vi "HFRR ADV v13.vi"() -> ()   [LabVIEW 2025] (continued)
                        n2641 = property on="Humidity ( %RH )" class="WFChart (strict)"("History Data"=w3931) -> ()  [unwired: 2 in, 2 out]
                        n2642 = property on="Stroke ( mm )" class="WFChart (strict)"("History Data"=w3932) -> ()  [unwired: 2 in, 2 out]
                        n2643 = property on="Temperature ( Deg C )" class="WFChart (strict)"("History Data"=w3931) -> ()  [unwired: 2 in, 2 out]
                        n2644 = property on="Service Password Log" class="Str"("Visible"=w3933) -> ()  [unwired: 2 in, 2 out]
                        n2645 = property on="Password 3" class="Clust (strict)"("Visible"=w3933) -> ()  [unwired: 2 in, 2 out]
                      }
                    }
                    "TEST FILE NAM,E SAVED" <- TRUE ("TEST FILE NAM,E SAVED")
                  }
                }
              }
            }
          }
        }
        n2646 = case shown="True" w3205 {
          frame False {
            n2647 = local write "tfalg"(0.0 ("tfalg")) -> ()
          }
          frame True {
            n2648 = local read "tfalg"() -> (w3350:dbl)
            n2649 = Equal?(x=w3350, y=0.0) -> (x = y?=w3351:bool)
            n2650 = case shown="True" w3351 {
              frame False {
              }
              frame True {
                n2651 = local read "Total No. of Tests"() -> (w3354:dbl)
                n2652 = local write "tfalg"(1.0 ("tfalg")) -> ()
                n2653 = local write "acq 2"(FALSE ("acq 2")) -> ()
                n2654 = Wait (ms)(milliseconds to wait=u32 200) -> ()  [unwired: 1 out]
                n2655 = Increment(x=w3354) -> (x+1=w3353:dbl)
                n2656 = local write "Total No. of Tests"(w3353) -> ()
              }
            }
          }
        }
        n2657 = local write "Test \nStatus"(w3211) -> ()
        n2658 = local write "st enable"(w3211) -> ()
        n2659 = local write "PWR"(w3211) -> ()
        n2660 = local write "Save"(w3211) -> ()
        n2661 = local read "Main Tab"() -> (w3168:T2)
        n2662 = case shown="True" w3192 {
          tunnel: [FALSE ("RUN") TRUE ("RUN")] -> w3191
          tunnel: [_ 1] -> w3184
          frame False {
          }
          frame True {
          }
        }
        n2663 = In Range and Coerce(upper limit=w3199, x=w3172, lower limit=w3198) -> (In Range?=w3190:bool)  [unwired: 1 out]
        n2664 = In Range and Coerce(upper limit=w3196, x=w3171, lower limit=w3197) -> (In Range?=w3188:bool)  [unwired: 1 out]
        n2665 = case shown="True" w3204 {
          frame False {
            n2666 = local read "Rt 3"() -> (w3332:bool)
            n2667 = case shown="True" w3332 {
              frame False {
              }
              frame True {
                n2668 = local write "Rt 3"(FALSE ("Rt 3")) -> ()
                n2669 = local write "Json End Flg"(TRUE ("Upld AR 2")) -> ()
              }
            }
            "Rt" <- TRUE ("Rt")
            "Rt 2" <- FALSE ("Rt")
          }
          frame True {
            n2670 = local read "Rt"() -> (w3339:bool)
            n2671 = local write "Rt 2"(TRUE ("Rt 2")) -> ()
            n2672 = case shown="True" w3339 {
              frame False {
              }
              frame True {
                w3340 = TRUE ("Upld AR 2")
                n2673 = local write "Rt"(FALSE ("Rt")) -> ()
                n2674 = local write "Upld AR"(w3340) -> ()
                n2675 = local write "Json St Flg"(w3340) -> ()
              }
            }
            "Rt 3" <- TRUE ("Rt 3")
          }
        }
        n2676 = case shown="True" w3190 {
          tunnel: [FALSE ("RUN") TRUE ("RUN")] -> w3189
          tunnel: [_ 2] -> w3183
          frame False {
          }
          frame True {
          }
        }
        n2677 = case shown="True" w3188 {
          tunnel: [FALSE ("RUN") TRUE ("RUN")] -> w3187
          tunnel: [_ 3] -> w3182
          frame False {
          }
          frame True {
          }
        }
        n2678 = case shown="\"Acquire\"" w3168 {
          tunnel: w3170 -> [_ w3401]
          frame Default {
            w3400 = 0.0 ("output")
            n2679 = local write "PID-out"(w3400) -> ()
            n2680 = local write "Frequency ( Hz )"(w3400) -> ()
          }
          frame "Acquire" {
            n2681 = stacked-sequence {
              frame #0 {
                n2682 = local read "Auto Start Test"() -> (w3403:bool)
                n2683 = case shown="True" w3403 {
                  tunnel: "RUN" -> [w3424 w3427]
                  tunnel: [w3424 w3426] -> w3404
                  frame False {
                  }
                  frame True {
                    n2684 = local read "Auto Start Temp"() -> (w3425:bool)
                    n2685 = Or(x=w3427, y=w3425) -> (x .or. y?=w3426:bool)
                  }
                }
                n2686 = local read "clk"() -> (w3423:dbl)
                n2687 = local read "Save"() -> (w3419:bool)
                n2688 = Equal?(x=w3423, y=0.0) -> (x = y?=w3420:bool)
                n2689 = And(x=w3420, y=w3419) -> (x .and. y?=w3421:bool)
                n2690 = Not(x="Engage") -> (.not. x?=w3410:bool)
                n2691 = case shown="True" w3404 {
                  tunnel: [w3435 w3453] -> w3406
                  frame False {
                    w3435 = 0.0
                    n2692 = local read "Auto Start Test"() -> (w3431:bool)
                    n2693 = local write "Reinit PID"(TRUE) -> ()
                    n2694 = local write "Start Time"(TRUE ("Start Time")) -> ()
                    n2695 = property on="Stroke" class="DigNum (strict)"("Visible"=TRUE) -> ()  [unwired: 2 in, 2 out]
                    n2696 = property on="Stroke 2" class="DigNum (strict)"("Visible"=FALSE) -> ()  [unwired: 2 in, 2 out]
                    n2697 = case shown="False" w3431 {
                      frame False {
                        n2698 = property on="Heater Button" class="Bool (strict)"("DisabledEnum"=T16."Enabled" ("Disabled")) -> ()  [unwired: 2 in, 2 out]
                        n2699 = property on="Humidity" class="Bool (strict)"("DisabledEnum"=T16."Enabled" ("Disabled")) -> ()  [unwired: 2 in, 2 out]
                      }
                      frame True {
                      }
                    }
                    n2700 = case shown="False" "TestCompFlg" {
                      frame False {
                        n2701 = local read "StartFlg"() -> (w3441:bool)
                        n2702 = case shown="True" w3441 {
                          frame False {
                          }
                          frame True {
                            n2703 = flat-sequence {
                              frame #0 {
                                n2704 = local read "EVENT LOG"() -> (w3443:string)
                                n2705 = call "Event Log.vi"("Content"="Test was interrupted", "EVENT LOG"=w3443) -> ("EVENT LOG"=w3444:string)  [unwired: 8 in, 1 out]
                                n2706 = local write "EVENT LOG"(w3444) -> ()
                              }
                              frame #1 {
                                w3445 = FALSE ("StartFlg")
                                n2707 = local write "Heater Button"(w3445) -> ()
                                n2708 = local write "StartFlg"(w3445) -> ()
                                n2709 = local write "Humidity"(w3445) -> ()
                              }
                            }
                          }
                        }
                      }
                      frame True {
                      }
                    }
                    n2710 = local write "String 14"("Test will autostart once parameters reach the set value." ("String 14")) -> ()
                    n2711 = local write "Old Pid Val"(w3435) -> ()
                  }
                  frame True {
                    n2712 = property on="Stroke 2" class="DigNum (strict)"("Visible"=TRUE) -> ()  [unwired: 2 in, 2 out]
                    n2713 = property on="Stroke" class="DigNum (strict)"("Visible"=FALSE) -> ()  [unwired: 2 in, 2 out]
                    n2714 = property on="STOP 2" class="Bool (strict)"("Disabled"=u8 2) -> ()  [unwired: 2 in, 2 out]
                    n2715 = local write "String 14"(" Running....." ("String 14")) -> ()
                    n2716 = property on="Heater Button" class="Bool (strict)"("DisabledEnum"=T16."Disabled and Grayed Out" ("Disabled")) -> ()  [unwired: 2 in, 2 out]
                    n2717 = property on="Humidity" class="Bool (strict)"("DisabledEnum"=T16."Disabled and Grayed Out" ("Disabled")) -> ()  [unwired: 2 in, 2 out]
                    n2718 = local read "PID Ref"() -> (w3464:bool)
                    n2719 = case shown="True" w3464 {
                      tunnel: [w3470 w3486] -> w3463
                      frame False {
                        n2720 = local read "Old Pid Val"() -> (w3470:dbl)
                      }
                      frame True {
                        n2721 = local read "Set Hz"() -> (w3479:dbl)
                        n2722 = local read "Frequency"() -> (w3490:dbl)
                        n2723 = Add(x=w3479, y=10.0) -> (x+y=w3488:dbl)
                        n2724 = Add(x=w3479, y=-10.0 ("Offset")) -> (x+y=w3497:dbl)
                        n2725 = Add(x=w3479, y=-10.0) -> (x+y=w3489:dbl)
                        n2726 = In Range and Coerce(upper limit=w3488, x=w3490, lower limit=w3489) -> (coerced(x)=w3478:dbl)  [unwired: 1 out]
                        n2727 = Or(x="Reinit PID", y="Reinit PID") -> (x .or. y?=w3487:bool)
                        n2728 = Multiply(x=w3497, y=0.1 ("Gain")) -> (x*y=w3476:dbl)
                        n2729 = local read "Elapsed time"() -> (w3483:dbl)
                        n2730 = local read "SPEED OUT:"() -> (w3498:dbl)
                        n2731 = Add(x=w3476, y=1.5) -> (x+y=w3474:dbl)
                        n2732 = call-poly <vilib>:"PID.vi"("reinitialize? (F)"=w3487, "output range"=cluster{"output high":dbl, "output low":dbl} {"output high"=1.0, "output low"=-1.0}, "PID gains"=T13 {"proportional gain (Kc)"=0.0005, "integral time (Ti, min)"=0.001, "derivative time (Td, min)"=0.0} ("Motor PID"), "process variable"=w3478, "setpoint"=w3479) -> ("output"=w3477:dbl)  [unwired: 5 in, 1 out]
                        n2733 = Multiply(x=w3474, y=w3498) -> (x*y=w3473:dbl)
                        n2734 = Greater?(x=w3483, y=0.05) -> (0:w3482:bool)
                        n2735 = case shown="True" w3482 {
                          tunnel: w3477 -> [_ w3500]
                          tunnel: [0.0 ("output") w3500] -> w3480
                          frame False {
                          }
                          frame True {
                            n2736 = local write "Reinit PID"(FALSE ("Reinit PID")) -> ()
                          }
                        }
                        n2737 = Multiply(x=w3473, y=0.8) -> (x*y=w3472:dbl)
                        n2738 = Add(x=w3472, y=w3480) -> (x+y=w3485:dbl)
                        n2739 = flat-sequence {
                          tunnel: [w3503] -> w3486
                          tunnel: w3485 -> [w3503]
                          frame #0 {
                            n2740 = local write "PID Ref"(FALSE ("PID Ref")) -> ()
                          }
                        }
                      }
                    }
                    "Old Pid Val" <- w3463
                    n2741 = case shown="True" "Start Time" {
                      selector: "Start Time" -> [_ w3466]
                      frame False {
                      }
                      frame True {
                        n2742 = Not(x=w3466) -> (.not. x?=w3465:bool)
                        n2743 = local write "Start Time"(w3465) -> ()
                        n2744 = local read "EVENT LOG"() -> (w3467:string)
                        n2745 = call "Event Log.vi"("Content"="Test in progress", "EVENT LOG"=w3467) -> ("EVENT LOG"=w3469:string)  [unwired: 8 in, 1 out]
                        n2746 = local write "EVENT LOG"(w3469) -> ()
                      }
                    }
                    n2747 = local read "Set Hz"() -> (w3460:dbl)
                    n2748 = call <vilib>:"Uniform White Noise Waveform.vi"() -> ("signal out"=w3459:waveform(dbl))  [unwired: 10 in, 1 out]
                    n2749 = local read "Freq"() -> (w3452:dbl)
                    n2750 = Add(x=w3460, y=w3459) -> (x+y=w3458:waveform(dbl))
                    n2751 = Multiply(x=w3458, y=ext 0.1) -> (x*y=w3454:waveform(ext))
                    n2752 = Multiply(x=w3452, y=0.9) -> (x*y=w3455:dbl)
                    n2753 = Add(x=w3454, y=w3455) -> (x+y=w3453:waveform(ext))
                    "StartFlg" <- TRUE ("StartFlg")
                  }
                }
                n2754 = case shown="True" w3421 {
                  frame False {
                  }
                  frame True {
                    n2755 = local write "clk"(10.0 ("clk")) -> ()
                    n2756 = Get Date/Time In Seconds() -> (seconds since 1Jan1904=w3506:timestamp)
                    n2757 = To Double Precision Float(number=w3506) -> (double precision float=w3504:dbl)
                    n2758 = local write "acq timer"(w3504) -> ()
                    n2759 = local write "act save time"(w3504) -> ()
                  }
                }
                n2760 = call "Elapsed Time"("Time Target (s)"="Countdown", "Reset"=w3410) -> ("Elapsed Time (s)"=w3415:dbl, "Time has Elapsed"=w3413:bool)  [unwired: 10 in, 6 out]
                "Countdown 2" <- w3415
                n2761 = Subtract(x=w3415, y=2.0) -> (x-y=w3418:dbl)
                n2762 = Less?(x=w3418, y="Countdown") -> (x < y?=w3416:bool)
                n2763 = And(x=w3416, y=w3413) -> (x .and. y?=w3412:bool)
                n2764 = case shown="True" w3412 {
                  frame False {
                  }
                  frame True {
                    (unwired) dbl[] [] ("History Data")
                    n2765 = local write "Engage"(FALSE ("Engage")) -> ()
                    n2766 = local write "RUN"(TRUE ("RUN")) -> ()
                    n2767 = local read "Humidity ( %RH )"() -> (→"Rh Before":dbl)
                  }
                }
                n2768 = local read "Test \nStatus"() -> (w3408:bool)
                n2769 = Select(t=w3406, s=w3408, f=0.0) -> (s? t:f=w3407:dbl)
                n2770 = local write "Frequency ( Hz )"(w3407) -> ()
                n2771 = local write "Freq"(w3407) -> ()
              }
              frame #1 {
                w3529 = 1000000.0 ("x")
                # "Elapsed time\ncof\nstroke\nAir temp\nTemp\nHumidity"
                # "acq timer\n\nact save time"
                # "convert to microseconds"
                n2772 = local read "COUNT"() -> (w3512:i32)
                n2773 = local read "Rate"() -> (w3525:dbl)
                n2774 = Divide(x=w3529, y=w3525) -> (x/y=w3530:dbl)
                n2775 = Greater Or Equal?(x=w3512, y=250) -> (x >= y?=w3511:bool)
                n2776 = Get Date/Time In Seconds() -> (seconds since 1Jan1904=w3532:timestamp)
                n2777 = case shown="True" w3511 {
                  frame False {
                    n2778 = local read "COUNT"() -> (w3533:i32)
                    n2779 = Increment(x=w3533) -> (x+1=w3534:i32)
                    n2780 = local write "COUNT"(w3534) -> ()
                  }
                  frame True {
                    n2781 = local write "COUNT"(0 ("COUNT")) -> ()
                  }
                }
                n2782 = local read "Samplingtime 2"() -> (w3510:dbl)
                n2783 = local read "act save time"() -> (w3527:dbl)
                n2784 = Divide(x=w3530, y=w3529) -> (x/y=w3528:dbl)
                n2785 = To Double Precision Float(number=w3532) -> (double precision float=w3521:dbl)
                n2786 = Add(x=w3527, y=w3510) -> (x+y=w3526:dbl)
                n2787 = local read "acq timer"() -> (w3531:dbl)
                n2788 = local read "COUNT"() -> (w3514:i32)
                n2789 = Greater Or Equal?(x=w3521, y=w3526) -> (x >= y?=w3509:bool)
                n2790 = Multiply(x=w3528, y=w3514) -> (x*y=w3520:dbl)
                n2791 = Subtract(x=w3521, y=w3531) -> (x-y=w3523:dbl)
                n2792 = local read "Save"() -> (w3524:bool)
                n2793 = Add(x=w3523, y=w3520) -> (x+y=w3507:dbl)
                "Elapsed time 3" <- w3507
                n2794 = And(x=w3509, y=w3524) -> (x .and. y?=w3522:bool)
                n2795 = Divide(x=w3507, y=60.0) -> (x/y=w3518:dbl)
                n2796 = local read "Test \nStatus"() -> (w3508:bool)
                n2797 = local read "clk"() -> (w3515:dbl)
                n2798 = Equal?(x=w3515, y=10.0) -> (x = y?=w3517:bool)
                n2799 = case shown="True" w3522 {
                  tunnel: w3521 -> [_ w3636]
                  tunnel: [FALSE ("Boolean 2") TRUE ("Boolean 2")] -> _
                  frame False {
                  }
                  frame True {
                    w3583 = ";" ("Substring")
                    # "Pid out/\nFreq response value"
                    n2800 = local write "act save time"(w3636) -> ()
                    n2801 = local read "FILE"() -> (w3577:string)
                    n2802 = call "file check.vi"("file name in"=w3577) -> ("error out"=w3580:errorcluster, "file name out"=w3575:string)  [unwired: 9 in]
                    n2803 = call "FILE PATH CREATION.vi"("error in"=w3580, "FILE NAME :"=w3575) -> ("FILE OUT"=w3578:path)  [unwired: 8 in, 1 out]
                    n2804 = Concatenate Strings(w3575, ".dgf" ("Substring")) -> (w3579:string)
                    n2805 = local read "Set Strk"() -> (w3607:dbl)
                    n2806 = local read "Stroke"() -> (w3598:dbl)
                    n2807 = local read "FF 2"() -> (→"Frictional Force ( N )" →"Frictional Force ( N )":dbl)
                    n2808 = Build Path(base path=w3578, name or relative path=w3579) -> (appended path=w3574:path)
                    n2809 = Subtract(x=w3598, y=w3607) -> (x-y=w3604:dbl)
                    n2810 = local read "COF 2"() -> (w3589:dbl)
                    "cof" <- w3589
                    "Coefficient of Friction" <- w3589
                    "COF 4" <- w3589
                    "Coefficient of Friction" <- w3589
                    n2811 = Multiply(x=w3604, y=0.05) -> (x*y=w3606:dbl)
                    n2812 = local read "TEMP"() -> (w3593:dbl)
                    "Temp" <- w3593
                    "Temperature ( Deg C )" <- w3593
                    n2813 = Add(x=w3606, y=w3607) -> (x+y=w3587:dbl)
                    "Stroke Ln" <- w3587
                    "Disp" <- w3587
                    n2814 = local read "ecr"() -> (w3590:dbl)
                    "Electrical Contact Resistance ( % )" <- w3590
                    n2815 = local read "Humidity ( %RH )"() -> (w3592:dbl)
                    "Humidity ( %RH )" <- w3592
                    "Humidity ( %RH )" <- w3592
                    n2816 = local read "Frequency ( Hz )"() -> (w3600:dbl)
                    n2817 = local read "Elapsed time"() -> (w3629:dbl)
                    n2818 = disable-structure shown="Disabled" {
                      frame Disabled {
                        n2819 = local read "ecr 3"() -> ()  [unwired: 1 in]
                      }
                      frame Enabled {
                      }
                    }
                    n2820 = local read "AIR TEMP"() -> (w3597:dbl)
                    n2821 = local read "PID-out"() -> (w3603:dbl)
                    n2822 = local write "Temperature ( Deg C )"(w3593) -> ()
                    n2823 = Number To Fractional String(number=w3587, width (-)=i16 9 ("precision (6)"), precision (6)=i16 6) -> (F-format string=w3622:string)  [unwired: 1 in]
                    n2824 = Number To Fractional String(number=w3597, width (-)=i16 9 ("precision (6)"), precision (6)=i16 3) -> (F-format string=w3621:string)  [unwired: 1 in]
                    n2825 = Number To Fractional String(number=w3593, width (-)=i16 9 ("precision (6)"), precision (6)=i16 3) -> (F-format string=w3618:string)  [unwired: 1 in]
                    n2826 = Number To Fractional String(number=w3592, width (-)=i16 9 ("precision (6)"), precision (6)=i16 3) -> (F-format string=w3615:string)  [unwired: 1 in]
                    n2827 = Number To Fractional String(number=w3590, width (-)=i16 9 ("precision (6)"), precision (6)=i16 3) -> (F-format string=w3612:string)  [unwired: 1 in]
                    n2828 = Number To Fractional String(number=w3603, width (-)=i16 9 ("precision (6)"), precision (6)=i16 3) -> (F-format string=w3608:string)  [unwired: 1 in]
                    n2829 = Number To Fractional String(number=w3600, width (-)=i16 9 ("precision (6)"), precision (6)=i16 3) -> (F-format string=w3599:string)  [unwired: 1 in]
                    n2830 = Number To Fractional String(number=w3589, width (-)=i16 9 ("precision (6)"), precision (6)=i16 6) -> (F-format string=w3630:string)  [unwired: 1 in]
                    n2831 = Number To Fractional String(number=w3629, width (-)=i16 14 ("precision (6)"), precision (6)=i16 3) -> (F-format string=w3631:string)  [unwired: 1 in]
                    n2832 = Bundle("y"=1.02, w3587, "y"=0.98) -> (w3591:cluster{"y":dbl, dbl, "y":dbl})  [unwired: 1 in]
                    n2833 = Number To Fractional String(number="Ambient Humidity :", width (-)=i16 9 ("precision (6)"), precision (6)=i16 6) -> (F-format string=w3581:string)  [unwired: 1 in]
                    n2834 = local read "RUN"() -> (w3588:bool)
                    n2835 = case shown="True" w3588 {
                      tunnel: w3591 -> [_ w3641]
                      tunnel: w3587 -> [_ w3640]
                      tunnel: w3587 -> [_ w3639]
                      tunnel: w3587 -> [_ w3638]
                      frame False {
                      }
                      frame True {
                        "Stroke ( mm )" <- w3641
                        "Stroke ( mm )" <- w3641
                        "Stroke 4" <- w3640
                        "Stroke 3" <- w3639
                        "Stroke 2" <- w3638
                      }
                    }
                    n2836 = Concatenate Strings(w3631, w3583, w3630, w3583, w3622, w3583, w3621, w3583, w3618, w3583, w3615, w3583, w3612, w3583, w3608, w3583, w3599, w3583, w3581, "\r") -> (w3628:string)
                    n2837 = call <vilib>:"Write Characters To File.vi"("append to file? (new file:F)"=TRUE, "character string"=w3628, "file path (dialog if empty)"=w3574) -> ()  [unwired: 2 in, 1 out]
                    "refresh flag" <- TRUE ("refresh flag")
                  }
                }
                n2838 = case shown="True" w3508 {
                  tunnel: w3518 -> [_ w3544]
                  tunnel: w3523 -> [_ w3554]
                  tunnel: [0.0 w3550] -> _
                  tunnel: w3517 -> [_ w3549]
                  tunnel: [0.0 w3548] -> _
                  tunnel: w3507 -> [_ w3548]
                  tunnel: w3521 -> [w3537 _]
                  frame False {
                    n2839 = local write "acq timer"(w3537) -> ()
                    n2840 = local write "Test Duration Status"(0.0 ("Test Duration Status")) -> ()
                  }
                  frame True {
                    n2841 = local read "Set Hz"() -> (w3551:dbl)
                    n2842 = local write "Elapsed time"(w3544) -> ()
                    n2843 = local read "test time"() -> (w3543:dbl)
                    n2844 = Multiply(x=w3554, y=w3551) -> (x*y=w3553:dbl)
                    n2845 = case shown="False" w3549 {
                      tunnel: w3553 -> [w3555 _]
                      tunnel: [w3555 1.0] -> w3550
                      frame False {
                        n2846 = local write "Cycles elapsed"(w3555) -> ()
                      }
                      frame True {
                      }
                    }
                    n2847 = Greater?(x=w3544, y=w3543) -> (0:w3552:bool)
                    n2848 = Subtract(x=w3543, y=w3544) -> (x-y=w3542:dbl)
                    "time" <- w3542
                    n2849 = Multiply(x=w3542, y=60.0) -> (x*y=w3541:dbl)
                    n2850 = local write "Time Remaining"(w3541) -> ()
                    n2851 = local write "Remaining Time"(w3541) -> ()
                    n2852 = case shown="True" w3552 {
                      frame False {
                      }
                      frame True {
                        w3557 = T16."Enabled" ("Disabled")
                        w3561 = "" ("FILE")
                        w3562 = TRUE ("Visible")
                        n2853 = local write "Humidity"(FALSE ("Humidity")) -> ()
                        n2854 = local write "RUN"(FALSE ("OK Button 2")) -> ()
                        n2855 = local write "Heater Button"(FALSE ("Heater Button")) -> ()
                        n2856 = local write "Auto Start Test"(FALSE ("Auto Start Test")) -> ()
                        n2857 = local write "TestCompFlg"(TRUE ("StpFlg")) -> ()
                        n2858 = local read "Humidity ( %RH )"() -> (→"Rh After":dbl)
                        n2859 = property on="STOP 2" class="Bool (strict)"("Disabled"=u8 0) -> ()  [unwired: 2 in, 2 out]
                        n2860 = local read "EVENT LOG"() -> (w3567:string)
                        n2861 = call "Event Log.vi"("Content"="Test Completed", "EVENT LOG"=w3567) -> ("EVENT LOG"=w3566:string)  [unwired: 8 in, 1 out]
                        n2862 = property on="RUN" class="Bool (strict)"("Visible"=w3562) -> ()  [unwired: 2 in, 2 out]
                        n2863 = property on="Auto Start Test" class="Bool (strict)"("Visible"=w3562) -> ()  [unwired: 2 in, 2 out]
                        n2864 = local write "Batch Ref Num :"(w3561) -> ()
                        n2865 = local write "FILE"(w3561) -> ()
                        n2866 = local write "EVENT LOG"(w3566) -> ()
                        n2867 = local write "TEST FILE NAM,E SAVED"(FALSE ("TEST FILE NAM,E SAVED")) -> ()
                        n2868 = local write "Fuel Discription :"(w3561) -> ()
                        n2869 = local write "Remarks :"(w3561) -> ()
                        n2870 = local write "Main Dashboard Buttons"(T1."Imaging" ("Main Dashboard Buttons")) -> ()
                        n2871 = local write "Main Tab"(T2."Adv Scar" ("Main Tab")) -> ()
                        n2872 = property on="FRICVALZ 2" class="Bool (strict)"("DisabledEnum"=w3557) -> ()  [unwired: 2 in, 2 out]
                        n2873 = property on="FRICVALZ 3" class="Bool (strict)"("DisabledEnum"=w3557) -> ()  [unwired: 2 in, 2 out]
                        n2874 = property on="FRICVALZ 4" class="Bool (strict)"("DisabledEnum"=w3557) -> ()  [unwired: 2 in, 2 out]
                      }
                    }
                    n2875 = Divide(x=w3544, y=w3543) -> (x/y=w3547:dbl)
                    n2876 = Multiply(x=w3547, y=100.0) -> (x*y=w3545:dbl)
                    n2877 = local write "Test Duration Status"(w3545) -> ()
                  }
                }
              }
              frame #2 {
                n2878 = case shown="True" "Heater Button" {
                  tunnel: [0.0 ("output") w3665] -> w3642
                  frame False {
                    w3645 = TRUE ("tmpchk")
                    n2879 = local read "TEMP"() -> (w3646:dbl)
                    n2880 = local write "Temp ini"(w3646) -> ()
                    n2881 = local write "Reset 4"(w3645) -> ()
                    n2882 = local write "tmpchk"(w3645) -> ()
                    n2883 = local write "reinit"(TRUE ("reinit")) -> ()
                    n2884 = local write "manual temp log"(TRUE ("manual temp log")) -> ()
                  }
                  frame True {
                    # "Logic to turn off\nthe heater when \ntemp is not rising.\nTime - 60 sec\nDelta t- 5°c"
                    n2885 = local read "Temp ini"() -> (w3653:dbl)
                    n2886 = local read "Auto Start Test"() -> (w3649:bool)
                    n2887 = Less?(x=w3653, y=53.0) -> (x < y?=w3651:bool)
                    n2888 = case shown="False" w3649 {
                      frame False {
                        n2889 = local read "Set Temp"() -> (w3676:dbl)
                        n2890 = local read "TEMP"() -> (w3675:dbl)
                        n2891 = Subtract(x=w3676, y=w3675) -> (x-y=w3674:dbl)
                        n2892 = Absolute Value(x=w3674) -> (abs(x)=w3673:dbl)
                        n2893 = Less?(x=w3673, y=0.5) -> (x < y?=w3671:bool)
                        n2894 = case shown="True" w3671 {
                          tunnel: "manual temp log" -> [_ w3677]
                          frame False {
                          }
                          frame True {
                            n2895 = case shown="True" w3677 {
                              selector: w3677 -> [_ w3678]
                              frame False {
                              }
                              frame True {
                                # "#Event log"
                                n2896 = Not(x=w3678) -> (.not. x?=w3679:bool)
                                n2897 = local write "manual temp log"(w3679) -> ()
                                n2898 = local read "EVENT LOG"() -> (w3682:string)
                                n2899 = call "Event Log.vi"("Content"="Target Temperature reached", "EVENT LOG"=w3682) -> ("EVENT LOG"=w3681:string)  [unwired: 8 in, 1 out]
                                n2900 = local write "EVENT LOG"(w3681) -> ()
                              }
                            }
                          }
                        }
                      }
                      frame True {
                        n2901 = local write "manual temp log"(TRUE ("manual temp log")) -> ()
                      }
                    }
                    n2902 = And(x="tmpchk", y=w3651) -> (x .and. y?=w3654:bool)
                    n2903 = case shown="True" w3654 {
                      frame False {
                      }
                      frame True {
                        n2904 = call "Elapsed Time8"("Time Target (s)"=300.0, "Reset"="Reset 4") -> ("Time has Elapsed"=w3684:bool)  [unwired: 10 in, 7 out]
                        n2905 = flat-sequence {
                          tunnel: w3684 -> [_]
                          frame #0 {
                            n2906 = local write "Reset 4"(FALSE ("Reset 4")) -> ()
                          }
                        }
                        n2907 = case shown="True" w3684 {
                          frame False {
                          }
                          frame True {
                            n2908 = local read "Temp ini"() -> (w3691:dbl)
                            n2909 = Add(x=w3691, y=5.0) -> (x+y=w3689:dbl)
                            n2910 = local read "TEMP"() -> (w3692:dbl)
                            n2911 = Greater?(x=w3692, y=w3689) -> (0:w3690:bool)
                            n2912 = case shown="False" w3690 {
                              frame False {
                                n2913 = local write "Heater Button"(FALSE ("Heater Button")) -> ()
                              }
                              frame True {
                                n2914 = local write "tmpchk"(FALSE ("tmpchk")) -> ()
                              }
                            }
                          }
                        }
                      }
                    }
                    n2915 = local read "Set Temp"() -> (w3662:dbl)
                    n2916 = local read "TEMP"() -> (w3656:dbl)
                    n2917 = call-poly <vilib>:"PID.vi"("reinitialize? (F)"="reinit", "output range"="output range", "dt (s)"=-1.0, "PID gains"="Temp PID gains", "process variable"=w3656, "setpoint"=w3662) -> ("output"=w3659:dbl)  [unwired: 4 in, 1 out]
                    n2918 = Subtract(x=w3662, y=w3656) -> (x-y=w3664:dbl)
                    n2919 = Add(x=w3662, y=0.5) -> (x+y=w3660:dbl)
                    n2920 = Greater Or Equal?(x=w3656, y=w3660) -> ()  [unwired: 1 out]
                    n2921 = Select(t=0.0, s=FALSE, f=w3659) -> (s? t:f=w3658:dbl)
                    "PID output" <- w3658
                    n2922 = flat-sequence {
                      tunnel: w3658 -> [w3695]
                      tunnel: [w3695] -> w3665
                      frame #0 {
                        n2923 = local write "reinit"(FALSE ("reinit")) -> ()
                      }
                    }
                    n2924 = Bundle(w3664, "output"=w3658, "TEMP"=w3656) -> (→"gTEMP 3":cluster{dbl, "output":dbl, "TEMP":dbl})  [unwired: 1 in]
                  }
                }
                "PID-out" <- w3642
              }
              frame #3 {
                n2925 = local read "TEMP"() -> (w3697:dbl)
                n2926 = Greater Or Equal?(x=w3697, y="Set Temp 2") -> (x >= y?=w3702:bool)
                n2927 = case shown="True" w3702 {
                  tunnel: [FALSE TRUE] -> w3700
                  frame False {
                  }
                  frame True {
                  }
                }
                "Status 13" <- w3700
                n2928 = And(x=w3700, y="trip1 8") -> (x .and. y?=w3699:bool)
                n2929 = case shown="True" w3699 {
                  frame False {
                    n2930 = local write "Heater Trip Temp"(TRUE ("Heater Trip Temp")) -> ()
                  }
                  frame True {
                    w3705 = FALSE ("OK Button 2")
                    n2931 = case shown="True" "Heater Trip Temp" {
                      selector: "Heater Trip Temp" -> [_ w3707]
                      frame False {
                      }
                      frame True {
                        n2932 = Not(x=w3707) -> (.not. x?=w3706:bool)
                        n2933 = local read "EVENT LOG"() -> (w3710:string)
                        n2934 = local write "Heater Trip Temp"(w3706) -> ()
                        n2935 = call "Event Log.vi"("Content"="Heater Trip", "EVENT LOG"=w3710) -> ("EVENT LOG"=w3709:string)  [unwired: 8 in, 1 out]
                        n2936 = local write "EVENT LOG"(w3709) -> ()
                      }
                    }
                    n2937 = local write "RUN"(w3705) -> ()
                    n2938 = property on="Auto Start Test" class="Bool (strict)"("Value"=w3705) -> ()  [unwired: 2 in, 2 out]
                    n2939 = local write "Heater Button"(w3705) -> ()
                  }
                }
              }
            }
            n2940 = case shown="False" w3401 {
              frame False {
                n2941 = disable-structure shown="Enabled" {
                  frame Enabled {
                    n2942 = stacked-sequence {
                      frame #0 {
                        n2943 = local write "RUN"(FALSE ("OK Button 2")) -> ()
                      }
                      frame #1 {
                      }
                    }
                  }
                  frame Disabled {
                  }
                }
              }
              frame True {
              }
            }
          }
        }
        n2944 = local read "airtempflg"() -> (w3193:bool)
        n2945 = Or(x=w3193, y=w3191) -> (x .or. y?=w3194:bool)
        n2946 = Insert Into Array(array=string[] ["Air Temperature has reached set value,", "Humidity has reached set value,", "Sample Temperaturehas reached set value,", ""], index=0, new element="") -> (w3179:string[])
        n2947 = Build Array(w3184, w3183, w3182) -> (w3180:i32[])
        n2948 = disable-structure shown="Disabled" {
          disable-tunnel: w3194 -> [w3271 _]
          disable-tunnel: w3189 -> [w3270 _]
          disable-tunnel: w3187 -> [w3269 _]
          frame Disabled {
            n2949 = Compound Arithmetic op=AND(w3271, w3270, w3269) -> ()  [unwired: 1 out]
            n2950 = case shown="True" {
              selector: _ -> [_ _]
              frame False {
              }
              frame True {
                w3272 = FALSE ("autostrtflg")
                n2951 = local write "RUN"(TRUE ("RUN")) -> ()
                n2952 = local write "autostrtflg"(w3272) -> ()
                n2953 = local write "autostart"(w3272) -> ()
                n2954 = local write "String 14"(" Running....." ("String 14")) -> ()
              }
            }
          }
          frame Enabled {
          }
        }
        n2955 = for {
          tunnel: w3180 -> [w3322] mode=indexing
          tunnel: w3179 -> [w3321]
          shift-right: [w3318] -> w3178
          shift-left: "" -> [w3320]
          n2956 = Index Array(array=w3321, index=w3322) -> (element=w3319:string)
          n2957 = Concatenate Strings(w3319, w3320) -> (w3318:string)
        }
        n2958 = local write "autostart 2"(w3178) -> ()
        n2959 = local read "Reset Graph"() -> (w3167:bool)
        n2960 = case shown="True" w3167 {
          selector: w3167 -> [_ w3221]
          frame False {
          }
          frame True {
            w3235 = 0.0 ("X Scale.Range:Maximum")
            n2961 = Not(x=w3221) -> (.not. x?=w3220:bool)
            n2962 = local write "Reset Graph"(w3220) -> ()
            n2963 = property on="Electrical Contact Resistance ( % )" class="WFChart (strict)"("XScale.Maximum"=600.0 ("X Scale.Range:Maximum"), "XScale.Minimum"=0.0 ("X Scale.Range:Minimum"), "YScale.Maximum"=100.0 ("Y Scale.Range:Maximum"), "YScale.Minimum"=0.0 ("Y Scale.Range:Minimum")) -> ()  [unwired: 2 in, 2 out]
            n2964 = property on="Frictional Force ( N )" class="WFChart (strict)"("XScale.Maximum"=600.0 ("X Scale.Range:Maximum"), "XScale.Minimum"=0.0 ("X Scale.Range:Minimum"), "YScale.Maximum"=100.0 ("Y Scale.Range:Maximum"), "YScale.Minimum"=0.0 ("Y Scale.Range:Minimum")) -> ()  [unwired: 2 in, 2 out]
            n2965 = property on="Temperature ( Deg C )" class="WFChart (strict)"("XScale.Maximum"=600.0 ("X Scale.Range:Maximum"), "XScale.Minimum"=0.0 ("X Scale.Range:Minimum"), "YScale.Maximum"=100.0 ("Y Scale.Range:Maximum"), "YScale.Minimum"=0.0 ("Y Scale.Range:Minimum")) -> ()  [unwired: 2 in, 2 out]
            n2966 = property on="Humidity ( %RH )" class="WFChart (strict)"("XScale.Maximum"=600.0 ("X Scale.Range:Maximum"), "XScale.Minimum"=0.0 ("X Scale.Range:Minimum"), "YScale.Maximum"=100.0 ("Y Scale.Range:Maximum"), "YScale.Minimum"=0.0 ("Y Scale.Range:Minimum")) -> ()  [unwired: 2 in, 2 out]
            n2967 = property on="Stroke ( mm )" class="WFChart (strict)"("XScale.Maximum"=600.0 ("X Scale.Range:Maximum"), "XScale.Minimum"=0.0 ("X Scale.Range:Minimum"), "YScale.Maximum"=100.0 ("Y Scale.Range:Maximum"), "YScale.Minimum"=0.0 ("Y Scale.Range:Minimum")) -> ()  [unwired: 2 in, 2 out]
            n2968 = property on="Coefficient of Friction" class="WFChart (strict)"("XScale.Maximum"=600.0 ("X Scale.Range:Maximum"), "XScale.Minimum"=0.0 ("X Scale.Range:Minimum"), "YScale.Maximum"=100.0 ("Y Scale.Range:Maximum"), "YScale.Minimum"=0.0 ("Y Scale.Range:Minimum")) -> ()  [unwired: 2 in, 2 out]
            n2969 = property on="Electrical Contact Resistance ( % )" class="WFChart (strict)"("XScale.Minimum"=0.0 ("X Scale.Range:Minimum"), "XScale.Maximum"=600.0 ("X Scale.Range:Maximum"), "YScale.Minimum"=0.0 ("Y Scale.Range:Minimum"), "YScale.Maximum"=100.0 ("Y Scale.Range:Maximum")) -> ()  [unwired: 2 in, 2 out]
            n2970 = property on="Temperature ( Deg C )" class="WFChart (strict)"("XScale.Minimum"=0.0 ("X Scale.Range:Minimum"), "XScale.Maximum"=600.0 ("X Scale.Range:Maximum"), "YScale.Minimum"=0.0 ("Y Scale.Range:Minimum"), "YScale.Maximum"=100.0 ("Y Scale.Range:Maximum")) -> ()  [unwired: 2 in, 2 out]
            n2971 = property on="Coefficient of Friction" class="WFChart (strict)"("XScale.Minimum"=0.0 ("X Scale.Range:Minimum"), "XScale.Maximum"=600.0 ("X Scale.Range:Maximum"), "YScale.Maximum"=1.0 ("X Scale.Range:Minimum"), "YScale.Minimum"=0.0 ("X Scale.Range:Minimum")) -> ()  [unwired: 2 in, 2 out]
            n2972 = property on="Frictional Force ( N )" class="WFChart (strict)"("XScale.Maximum"=600.0 ("X Scale.Range:Maximum"), "XScale.Minimum"=w3235, "YScale.Maximum"=10.0 ("Y Scale.Range:Maximum"), "YScale.Minimum"=w3235) -> ()  [unwired: 2 in, 2 out]
            n2973 = property on="Stroke ( mm )" class="WFChart (strict)"("XScale.Maximum"=600.0 ("X Scale.Range:Maximum"), "XScale.Minimum"=0.0 ("X Scale.Range:Minimum"), "YScale.Maximum"=100.0 ("Y Scale.Range:Maximum"), "YScale.Minimum"=0.0 ("Y Scale.Range:Minimum")) -> ()  [unwired: 2 in, 2 out]
            n2974 = property on="Humidity ( %RH )" class="WFChart (strict)"("XScale.Maximum"=600.0 ("X Scale.Range:Maximum"), "XScale.Minimum"=0.0 ("X Scale.Range:Minimum"), "YScale.Maximum"=100.0 ("Y Scale.Range:Maximum"), "YScale.Minimum"=0.0 ("Y Scale.Range:Minimum")) -> ()  [unwired: 2 in, 2 out]
          }
        }
      }
      frame "Compare Files" {
        # "Elapsed time\ncof\nstroke\nAir temp\nTemp\nHumidity"
        n2975 = case shown="True" "RSTV1 2" {
          frame False {
          }
          frame True {
            n2976 = property on="Humidity ( %RH )" class="XYGraph (strict)"("Y Scale.Display Format:Precision"=u8 0 ("Y Scale.Format & Precision:Precision")) -> ()  [unwired: 2 in, 2 out]
            n2977 = property on="Humidity ( %RH )" class="XYGraph (strict)"("X Scale.Range:Minimum"=0.0, "X Scale.Range:Maximum"=75.0, "Y Scale.Range:Minimum"=48.0, "Y Scale.Range:Maximum"=58.0) -> ()  [unwired: 2 in, 2 out]
          }
        }
        n2978 = case shown="True" "RST CP 2" {
          frame False {
          }
          frame True {
            n2979 = property on="XY Graph 13" class="XYGraph (strict)"("Y Scale.Display Format:Precision"=u8 0 ("Y Scale.Format & Precision:Precision")) -> ()  [unwired: 2 in, 2 out]
            n2980 = property on="XY Graph 13" class="XYGraph (strict)"("X Scale.Range:Minimum"=0.0, "X Scale.Range:Maximum"=75.0, "Y Scale.Range:Minimum"=0.0, "Y Scale.Range:Maximum"=100.0) -> ()  [unwired: 2 in, 2 out]
          }
        }
        n2981 = case shown="True" "RST CP" {
          frame False {
          }
          frame True {
            n2982 = property on="Sample Temperature ( °C )" class="XYGraph (strict)"("Y Scale.Display Format:Precision"=u8 2 ("Y Scale.Format & Precision:Precision")) -> ()  [unwired: 2 in, 2 out]
            n2983 = property on="Sample Temperature ( °C )" class="XYGraph (strict)"("X Scale.Range:Minimum"=0.0, "X Scale.Range:Maximum"=75.0, "Y Scale.Range:Minimum"=58.0, "Y Scale.Range:Maximum"=62.0) -> ()  [unwired: 2 in, 2 out]
          }
        }
        n2984 = case shown="True" "RSTV1 3" {
          frame False {
          }
          frame True {
            n2985 = property on="Air Temperature  ( °C )" class="XYGraph (strict)"("Y Scale.Display Format:Precision"=u8 2 ("Y Scale.Format & Precision:Precision")) -> ()  [unwired: 2 in, 2 out]
            n2986 = property on="Air Temperature  ( °C )" class="XYGraph (strict)"("X Scale.Range:Minimum"=0.0 ("Y Scale.Range:Minimum"), "X Scale.Range:Maximum"=75.0 ("Y Scale.Range:Maximum"), "Y Scale.Range:Minimum"=20.0 ("X Scale.Range:Minimum"), "Y Scale.Range:Maximum"=26.0 ("X Scale.Range:Maximum")) -> ()  [unwired: 2 in, 2 out]
          }
        }
        n2987 = case shown="True" "RSTV1 4" {
          frame False {
          }
          frame True {
            n2988 = property on="Stroke ( mm )" class="XYGraph (strict)"("Y Scale.Display Format:Precision"=u8 2 ("Y Scale.Format & Precision:Precision")) -> ()  [unwired: 2 in, 2 out]
            n2989 = property on="Stroke ( mm )" class="XYGraph (strict)"("X Scale.Range:Minimum"=0.0 ("Y Scale.Range:Maximum"), "X Scale.Range:Maximum"=75.0 ("X Scale.Range:Minimum"), "Y Scale.Range:Minimum"=0.98, "Y Scale.Range:Maximum"=1.02) -> ()  [unwired: 2 in, 2 out]
          }
        }
        n2990 = case shown="True" "rstv2" {
          frame False {
          }
          frame True {
            n2991 = property on="Coefficient Of Friction" class="XYGraph (strict)"("Y Scale.Display Format:Precision"=u8 3 ("Y Scale.Format & Precision:Precision")) -> ()  [unwired: 2 in, 2 out]
            n2992 = property on="Coefficient Of Friction" class="XYGraph (strict)"("X Scale.Range:Minimum"=0.0 ("Y Scale.Range:Maximum"), "X Scale.Range:Maximum"=75.0, "Y Scale.Range:Minimum"=0.0, "Y Scale.Range:Maximum"=1.0 ("X Scale.Range:Minimum")) -> ()  [unwired: 2 in, 2 out]
          }
        }
        n2993 = case shown="True" "RST CP 3" {
          frame False {
          }
          frame True {
            n2994 = property on="Air Temp ( °C ) vs Humidity ( % RH )" class="XYGraph (strict)"("X Scale.Range:Minimum"=18.0, "X Scale.Range:Maximum"=28.0 ("X Scale.Range:Minimum"), "Y Scale.Range:Minimum"=30.0 ("X Scale.Range:Minimum"), "Y Scale.Range:Maximum"=70.0 ("X Scale.Range:Minimum")) -> ()  [unwired: 2 in, 2 out]
          }
        }
        n2995 = case shown="True" "OPEN 1" {
          frame False {
          }
          frame True {
            (unwired) 0  # existing file
            w3986 = "Choose a datalog file to open"  # prompt
            n2996 = local write "OPEN 1"(FALSE ("OPEN 1")) -> ()
            n2997 = String To Path(string="C:\\LAB-IQ\\Data\\") -> (path=w3971:path)
            n2998 = File Dialog(6:"*.dgf" ("pattern"), 7:w3986, 11:w3971) -> (0:w3969:errorcluster, 3:w3977:path)  [unwired: 4 in, 2 out]
            n2999 = Unbundle(w3969) -> ()  [unwired: 3 out]
            n3000 = Strip Path(path=w3977) -> (name=w3976:string)  [unwired: 1 out]
            n3001 = Path To String(path=w3977) -> (string=w3972:string)
            "string1" <- w3972
            n3002 = Match Pattern(string=w3976, regular expression=".dgf") -> (before substring=→"String Control":string)  [unwired: 1 in, 3 out]
            n3003 = Match Pattern(string=w3972, regular expression=".dgf" ("substring (\"\")")) -> (before substring=w3982:string)  [unwired: 1 in, 3 out]
            n3004 = Concatenate Strings(w3982, ".duf" ("Substring")) -> (w3978:string)
            n3005 = String To Path(string=w3978) -> (path=w3983:path)
            n3006 = call <vilib>:"Read Characters From File.vi"("file path (dialog if empty)"=w3983, "start of read offset (chars.:0)"=60 ("start of read offset (chars.: 0)")) -> ("character string"=→"String Control 2":string)  [unwired: 4 in, 3 out]
          }
        }
        n3007 = case shown="True" "OPEN 2" {
          frame False {
          }
          frame True {
            (unwired) 0  # existing file
            w4004 = "Choose a datalog file to open"  # prompt
            n3008 = local write "OPEN 2"(FALSE ("OPEN 1")) -> ()
            n3009 = String To Path(string="C:\\LAB-IQ\\Data\\") -> (path=w3989:path)
            n3010 = File Dialog(6:"*.dgf" ("pattern"), 7:w4004, 11:w3989) -> (0:w3987:errorcluster, 3:w3995:path)  [unwired: 4 in, 2 out]
            n3011 = Unbundle(w3987) -> ()  [unwired: 3 out]
            n3012 = Strip Path(path=w3995) -> (name=w3993:string)  [unwired: 1 out]
            n3013 = Path To String(path=w3995) -> (string=w3990:string)
            "string1 2" <- w3990
            n3014 = Match Pattern(string=w3993, regular expression=".dgf") -> (before substring=→"String Control 3":string)  [unwired: 1 in, 3 out]
            n3015 = Match Pattern(string=w3990, regular expression=".dgf" ("substring (\"\")")) -> (before substring=w4001:string)  [unwired: 1 in, 3 out]
            n3016 = Concatenate Strings(w4001, ".duf" ("Substring")) -> (w3998:string)
            n3017 = String To Path(string=w3998) -> (path=w3996:path)
            n3018 = call <vilib>:"Read Characters From File.vi"("file path (dialog if empty)"=w3996, "start of read offset (chars.:0)"=60 ("start of read offset (chars.: 0)")) -> ("character string"=→"String Control 4":string)  [unwired: 4 in, 3 out]
          }
        }
        n3019 = case shown="True" "OPEN 3" {
          frame False {
          }
          frame True {
            (unwired) 0  # existing file
            w4022 = "Choose a datalog file to open"  # prompt
            n3020 = local write "OPEN 3"(FALSE ("OPEN 1")) -> ()
            n3021 = String To Path(string="C:\\LAB-IQ\\Data\\") -> (path=w4007:path)
            n3022 = File Dialog(6:"*.dgf" ("pattern"), 7:w4022, 11:w4007) -> (0:w4005:errorcluster, 3:w4013:path)  [unwired: 4 in, 2 out]
            n3023 = Unbundle(w4005) -> ()  [unwired: 3 out]
            n3024 = Strip Path(path=w4013) -> (name=w4011:string)  [unwired: 1 out]
            n3025 = Path To String(path=w4013) -> (string=w4008:string)
            "string1 3" <- w4008
            n3026 = Match Pattern(string=w4011, regular expression=".dgf") -> (before substring=→"String Control 5":string)  [unwired: 1 in, 3 out]
            n3027 = Match Pattern(string=w4008, regular expression=".dgf" ("substring (\"\")")) -> (before substring=w4018:string)  [unwired: 1 in, 3 out]
            n3028 = Concatenate Strings(w4018, ".duf" ("Substring")) -> (w4015:string)
            n3029 = String To Path(string=w4015) -> (path=w4019:path)
            n3030 = call <vilib>:"Read Characters From File.vi"("file path (dialog if empty)"=w4019, "start of read offset (chars.:0)"=60 ("start of read offset (chars.: 0)")) -> ("character string"=→"String Control 6":string)  [unwired: 4 in, 3 out]
          }
        }
        n3031 = case shown="True" "OPEN 4" {
          frame False {
          }
          frame True {
            (unwired) 0  # existing file
            w4040 = "Choose a datalog file to open"  # prompt
            n3032 = local write "OPEN 4"(FALSE ("OPEN 1")) -> ()
            n3033 = String To Path(string="C:\\LAB-IQ\\Data\\") -> (path=w4025:path)
            n3034 = File Dialog(6:"*.dgf" ("pattern"), 7:w4040, 11:w4025) -> (0:w4023:errorcluster, 3:w4031:path)  [unwired: 4 in, 2 out]
            n3035 = Unbundle(w4023) -> ()  [unwired: 3 out]
            n3036 = Strip Path(path=w4031) -> (name=w4029:string)  [unwired: 1 out]
            n3037 = Path To String(path=w4031) -> (string=w4026:string)
            "string1 4" <- w4026
            n3038 = Match Pattern(string=w4029, regular expression=".dgf") -> (before substring=→"String Control 7":string)  [unwired: 1 in, 3 out]
            n3039 = Match Pattern(string=w4026, regular expression=".dgf" ("substring (\"\")")) -> (before substring=w4036:string)  [unwired: 1 in, 3 out]
            n3040 = Concatenate Strings(w4036, ".duf" ("Substring")) -> (w4033:string)
            n3041 = String To Path(string=w4033) -> (path=w4037:path)
            n3042 = call <vilib>:"Read Characters From File.vi"("file path (dialog if empty)"=w4037, "start of read offset (chars.:0)"=60 ("start of read offset (chars.: 0)")) -> ("character string"=→"String Control 8":string)  [unwired: 4 in, 3 out]
          }
        }
      }
      frame "About" {
        # "Elapsed time\ncof\nstroke\nmean pos\nTemp\nHumidity"
        n3043 = disable-structure shown="Disabled" {
          frame Disabled {
            n3044 = case shown="True" "Export" {
              frame False {
              }
              frame True {
                w4062 = "                                      " ("string")
                w4064 = "\r"
                (unwired) i16 6 ("width (-)")
                w4141 = "\r"
                w4073 = "\r"
                n3045 = local write "Export"(FALSE ("Export")) -> ()
                n3046 = local read "String 29"() -> (w4110:string)
                n3047 = local read "String 34"() -> (w4098:string)
                n3048 = local read "String 35"() -> (w4093:string)
                n3049 = local read "String 37"() -> (w4089:string)
                n3050 = local read "String 36"() -> (w4086:string)
                n3051 = local read "String 38"() -> (w4083:string)
                n3052 = local read "String 39"() -> (w4080:string)
                n3053 = Match Pattern(string=w4110, regular expression=".dwm") -> (before substring=w4106:string)  [unwired: 1 in, 3 out]
                "before substring" <- w4106
                n3054 = local read "S 38"() -> (w4101:string)
                n3055 = local read "S 39"() -> (w4094:string)
                n3056 = local read "Temperature before test 2"() -> (w4130:dbl)
                n3057 = local read "Temperature after test 2"() -> (w4135:dbl)
                n3058 = local read "Humidity before test 2"() -> (w4116:dbl)
                n3059 = local read "Humidity after test 2"() -> (w4131:dbl)
                n3060 = local read "MWSD 2"() -> (w4127:dbl)
                n3061 = local read "WS1.4 2"() -> (w4143:dbl)
                n3062 = local read "HCF 2"() -> (w4139:dbl)
                n3063 = local read "AVP 2"() -> (w4128:dbl)
                n3064 = Concatenate Strings("1," ("string"), w4101) -> (w4100:string)
                n3065 = Concatenate Strings("2," ("string"), w4098) -> (w4097:string)
                n3066 = Concatenate Strings("3," ("string"), w4094) -> (w4096:string)
                n3067 = Concatenate Strings("4," ("string"), w4093) -> (w4092:string)
                n3068 = Concatenate Strings("5," ("string"), w4089) -> (w4090:string)
                n3069 = Concatenate Strings("6," ("string"), w4086) -> (w4087:string)
                n3070 = Concatenate Strings("7," ("string"), w4083) -> (w4084:string)
                n3071 = Concatenate Strings("8," ("string"), w4080) -> (w4081:string)
                n3072 = local read "Sample ID"() -> (w4148:string)
                n3073 = case shown="\"xlx\"" "Select File Type" {
                  tunnel: w4106 -> [w4151 w4153 w4155]
                  tunnel: [w4149 w4154 w4156] -> w4105
                  frame "xlx" {
                    n3074 = Concatenate Strings(w4151, ".xls" ("string")) -> (w4149:string)
                  }
                  frame "csv" {
                    n3075 = Concatenate Strings(w4153, ".csv" ("string")) -> (w4154:string)
                  }
                  frame "txt" {
                    n3076 = Concatenate Strings(w4155, ".txt" ("string")) -> (w4156:string)
                  }
                }
                n3077 = local read "Test Date"() -> (w4147:string)
                n3078 = local read "String 45"() -> (w4061:string)
                n3079 = local read "String 31"() -> (w4146:string)
                n3080 = local read "String 32"() -> (w4145:string)
                n3081 = local read "TITTLE"() -> (w4069:string)
                n3082 = Number To Fractional String(number=w4116, width (-)=i16 6, precision (6)=i16 2) -> (F-format string=w4115:string)  [unwired: 1 in]
                n3083 = Number To Fractional String(number=w4130, width (-)=i16 6, precision (6)=i16 2) -> (F-format string=w4136:string)  [unwired: 1 in]
                n3084 = Number To Fractional String(number=w4131, width (-)=i16 6, precision (6)=i16 2) -> (F-format string=w4129:string)  [unwired: 1 in]
                n3085 = Number To Fractional String(number=w4135, width (-)=i16 6, precision (6)=i16 2) -> (F-format string=w4134:string)  [unwired: 1 in]
                n3086 = Number To Fractional String(number=w4127, width (-)=i16 6, precision (6)=i16 2) -> (F-format string=w4125:string)  [unwired: 1 in]
                n3087 = Number To Fractional String(number=w4128, width (-)=i16 6, precision (6)=i16 2) -> (F-format string=w4126:string)  [unwired: 1 in]
                n3088 = Number To Fractional String(number=w4139, width (-)=i16 6, precision (6)=i16 2) -> (F-format string=w4140:string)  [unwired: 1 in]
                n3089 = Number To Fractional String(number=w4143, precision (6)=i16 2) -> (F-format string=w4144:string)  [unwired: 2 in]
                n3090 = local read "s.NO"() -> (w4063:string)
                n3091 = Concatenate Strings("=" ("string"), w4069) -> (w4068:string)
                n3092 = Concatenate Strings("S.No," ("string"), "                                       Parameters" ("string")) -> (w4074:string)
                n3093 = Concatenate Strings(w4141, w4100, w4115, w4141, w4097, w4136, w4141, w4096, w4129, w4141, w4092, w4134, w4141, w4090, w4125, w4141, w4087, w4126, w4141, w4084, w4140, w4141, w4081, w4144) -> (w4103:string)
                n3094 = Concatenate Strings(w4073, "," ("string"), w4061, w4063, w4062, w4145, w4148, w4062, w4146, w4147, w4073) -> (w4071:string)
                n3095 = local read "Tested by"() -> (w4077:string)
                n3096 = local read "String 33"() -> (w4078:string)
                n3097 = Concatenate Strings("," ("string"), "                                                                             " ("string")) -> (w4066:string)
                n3098 = Concatenate Strings(w4068, w4064, w4071, w4064, w4074, w4103, w4064, w4066, w4078, w4077) -> (→"export":string)
                n3099 = String To Path(string=w4105) -> (path=w4112:path)
                n3100 = local read "export"() -> (w4107:string)
                n3101 = call <vilib>:"Write Characters To File.vi"("append to file? (new file:F)"=FALSE, "character string"=w4107, "file path (dialog if empty)"=w4112) -> ()  [unwired: 2 in, 1 out]
              }
            }
          }
          frame Enabled {
          }
        }
        n3102 = case shown="True" "OK Button 17" {
          frame False {
          }
          frame True {
            (unwired) 0  # existing file
            w4365 = "Choose a datalog file to open"  # prompt
            n3103 = local write "OK Button 17"(FALSE ("OK Button 17")) -> ()
            n3104 = local read "String"() -> (w4360:string)
            n3105 = String To Path(string=w4360) -> (path=w4361:path)
            n3106 = File Dialog(6:"*.duf" ("pattern"), 7:w4365, 11:w4361) -> (0:w4352:errorcluster, 3:w4371:path)  [unwired: 4 in, 2 out]
            n3107 = Unbundle(w4352) -> ()  [unwired: 3 out]
            n3108 = Open/Create/Replace File "Open File"(file path (use dialog)=w4371) -> (refnum out=w4363:refnum<file>)  [unwired: 5 in, 2 out]
            n3109 = Strip Path(path=w4371) -> (name=w4369:string)  [unwired: 1 out]
            n3110 = Path To String(path=w4371) -> (string=w4354:string)
            n3111 = while {
              tunnel: w4363 -> [w4375]
              i -> [w4372]
              stop <- w4373 continue-if-true
              (unwired) TRUE ("line mode (F)")
              n3112 = Read from Text File "Read File"(file (use dialog)=w4375) -> (text=w4374:string)  [unwired: 3 in, 3 out]
              n3113 = local write "Numeric 16"(w4372) -> ()
              n3114 = String Length(string=w4374) -> (length=w4377:i32)
              n3115 = Greater?(x=w4377, y=1) -> (0:w4373:bool)
            }
            n3116 = local write "String 29"(w4354) -> ()
            n3117 = Search and Replace String(input string=w4354, search string=".duf", replace string=".dgf" ("replace string (\"\")")) -> (result string=→"String Indicator 4":string)  [unwired: 5 in, 3 out]
            n3118 = Match Pattern(string=w4369, regular expression=".dwm") -> (before substring=w4353:string)  [unwired: 1 in, 3 out]
            "String Indicator" <- w4353
            n3119 = Match Pattern(string=w4354, regular expression=".dwm" ("substring (\"\")")) -> (before substring=w4355:string)  [unwired: 1 in, 3 out]
            "String Indicator 3" <- w4355
            n3120 = local write "TITTLE 2"(w4353) -> ()
            n3121 = String To Path(string=w4355) -> (path=w4362:path)
            "path" <- w4362
            n3122 = call <vilib>:"Read Characters From File.vi"("file path (dialog if empty)"=w4362, "start of read offset (chars.:0)"=60 ("start of read offset (chars.: 0)")) -> ("character string"=→"String Indicator 2":string)  [unwired: 4 in, 3 out]
          }
        }
        n3123 = call <vilib>:"Query Available Printers.vi"() -> ("system configured printers"=w4054:string[])  [unwired: 9 in, 2 out]
        "System Configured Printers 2" <- w4054
        n3124 = local read "OK Button 16"() -> (w4051:bool)
        n3125 = case shown="True" "OK Button 16" {
          frame False {
          }
          frame True {
            n3126 = stacked-sequence {
              frame #0 {
                n3127 = local read "Numeric 16"() -> (w4379:i32)
                n3128 = local write "Numeric 10"(w4379) -> ()
              }
              frame #1 {
                n3129 = local read "S.NO"() -> (→"s.NO":string)
                n3130 = local read "String 29"() -> (w4383:string)
                n3131 = String To Path(string=w4383) -> (path=w4382:path)
                n3132 = Open/Create/Replace File "Open File"(file path (use dialog)=w4382) -> (refnum out=w4384:refnum<file>)  [unwired: 5 in, 2 out]
                n3133 = for {
                  N: 16 -> [_]
                  tunnel: w4384 -> [w4391]
                  i -> [w4387]
                  (unwired) TRUE ("line mode (F)")
                  n3134 = Read from Text File "Read File"(file (use dialog)=w4391) -> (text=w4385:string)  [unwired: 3 in, 3 out]
                  n3135 = Match Pattern(string=w4385, regular expression="(") -> (after substring=w4390:string)  [unwired: 1 in, 3 out]
                  n3136 = Match Pattern(string=w4390, regular expression=")") -> (before substring=w4386:string)  [unwired: 1 in, 3 out]
                  n3137 = case shown="1" w4387 {
                    tunnel: w4386 -> [w4392 w4393 _ _ w4394 w4395 w4396 w4398 w4400 w4402 w4404 w4406 w4408 w4410 _]
                    tunnel: w4385 -> [_ _ _ _ _ _ _ _ _ _ _ _ _ _ _]
                    frame 0 {
                      "TITTLE" <- w4392
                    }
                    frame 1 {
                      "Sample ID" <- w4393
                    }
                    frame 2 {
                    }
                    frame 3 {
                    }
                    frame 4 {
                      "Test Date" <- w4394
                    }
                    frame 5 {
                      "Tested by" <- w4395
                    }
                    frame 6 {
                      n3138 = Fract/Exp String To Number(string=w4396) -> (number=→"Humidity before test 2":dbl)  [unwired: 3 in, 1 out]
                    }
                    frame 7 {
